vi "ReadIniFile.vi"() -> ()   [LabVIEW 2014]
uses:
  Users/Chris Rogers/Desktop/VIOLIN/CurtinVIs/Code/DataControl.ctl
  Users/Chris Rogers/Desktop/VIOLIN/CurtinVIs/Code/SettingsControl.ctl
panel:
  out "App:Default Data Directory":path
  in  "Sample rate (Hz)":dbl(slide)=22050.0 min=8000.0 max=48000.0 scale=8000.0..48000.0
  in  "#Channels":i32(ring)=2 items=["1"=1, "2"=2]
  in  "Resolution (bits)":i32=16 min=1 max=32
  in  "Data":T1[](array[typedef]) {"Settings"."Time" format="%<%H:%M\n%d/%m/%y>T"}
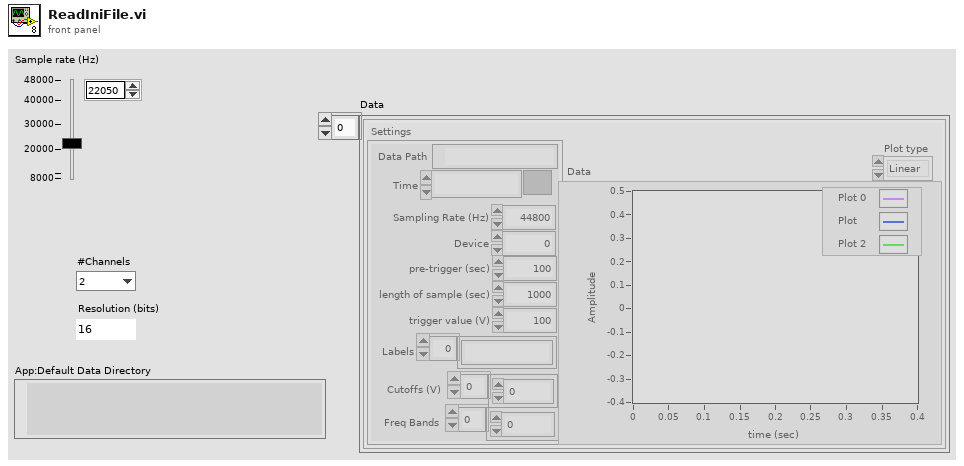
[diagram p1: front panel]
types:
  T1 = typedef "DataControl.ctl" = cluster{"Settings":T2, "Data":cluster{i32, dbl, "data":dbl[]}[], "Plot type":enum16{"Linear", "log"}}
  T2 = typedef "SettingsControl.ctl" = cluster{"Data Path":path, "Time":timestamp, "Sampling Rate (Hz)":u16, "Device":u16, "pre-trigger (sec)":dbl, "length of sample (sec)":dbl, "trigger value (V)":dbl, "Labels":string[], "Cutoffs (V)":dbl[], "Freq Bands":dbl[]}
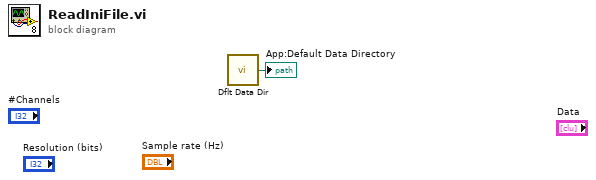
[diagram p0: block diagram]
diagram:
  n1 = call <vilib>:"Dflt Data Dir.vi"() -> ("App:Default Data Directory"=→"App:Default Data Directory":path)
